vi "UFF_ParseBytes.vi"(8 "length":i32, 11 "String in":string) -> (0 "number":dbl, 1 "Value":i32, 2 "Subset":string, 3 "String out":string, 4 "no error":bool)   [LabVIEW 2022 SP3]
uses:
  <vilib>/Utility/error.llb/Trim Whitespace One-Sided.vi
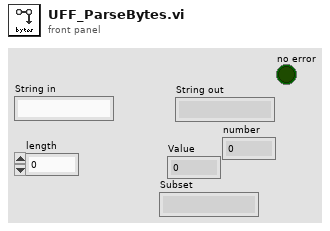
[diagram p1: front panel]
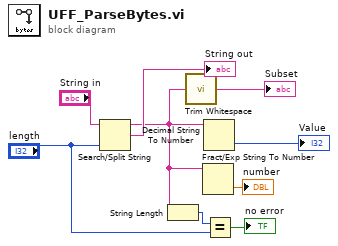
[diagram p0: block diagram]
diagram:
  n1 = Search/Split String(string="String in", offset (0)="length") -> (substring before match=w4:string, match + rest of string=→"String out":string)  [unwired: 1 in, 1 out]
  n2 = String Length(string=w4) -> (length=w3:i32)
  n3 = call <vilib>:"Trim Whitespace.vi"("string"=w4) -> ("trimmed string"=→"Subset":string)  [unwired: 1 in]
  n4 = Fract/Exp String To Number(string=w4) -> (number=→"number":dbl)  [unwired: 3 in, 1 out]
  n5 = Decimal String To Number(string=w4) -> (number=→"Value":i32)  [unwired: 2 in, 1 out]
  n6 = Equal?(x=w3, y="length") -> (x = y?=→"no error":bool)
